vi "设置延时.vi"(8 "error in (no error)":errorcluster caption="错误输入（无错误）", 11 "Simulation DMM 输入":refnum<class "Simulation DMM.lvclass">) -> (0 "error out":errorcluster caption="错误输出", 3 "Simulation DMM 输出":refnum<class "Simulation DMM.lvclass">)   [LabVIEW 2020, in "Simulation DMM.lvlib" / "Simulation DMM.lvclass"]
uses:
  Simulation DMM.lvclass
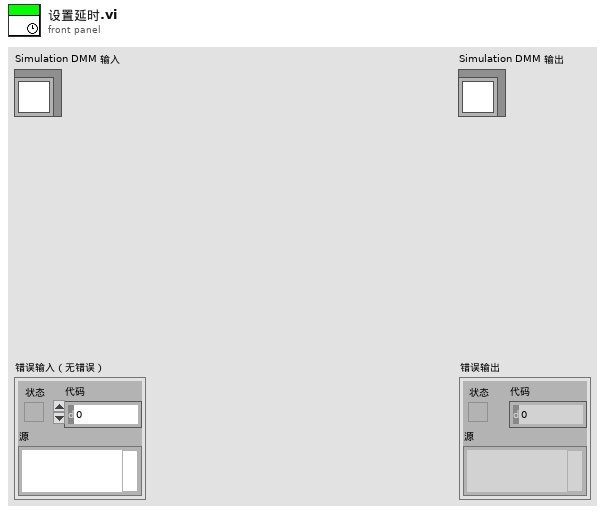
[diagram p1: front panel]
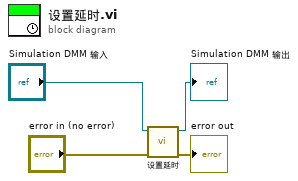
[diagram p0: block diagram]
diagram:
  n1 = call-parent "设置延时.vi"("error in (no error)"="error in (no error)", "数字多用表接口 输入"="Simulation DMM 输入") -> ("error out"=→"error out":errorcluster, "数字多用表接口 输出"=→"Simulation DMM 输出":refnum<class "Simulation DMM.lvclass">)  [unwired: 8 in]
